vi "MPExxx_Reset.vi"(2 "error in (no error)":errorcluster, 3 "VISA session":refnum<visa-resource-name>) -> (0 "error out":errorcluster, 1 "dup VISA session":refnum<visa-resource-name>)   [LabVIEW 2023]
doc: "This command resets the power supply to factory default states as defined below.\n\n OUTP[:STAT] OFF\n CURR[:LEV][:IMM] 0 \n CURR[:LEV]:TRIG 0 \n VOLT[:LEV][:IMM] 0 \n VOLT[:LEV]:TRIG 0 \n PER 0\n INIT:CONT OFF\n VOLT:PROT[:LEV] 110% of MAX\n CURR:PROT[:LEV] 110% of MAX"
panel:
  # "MAGNA-POWER"
  # "Electronics"
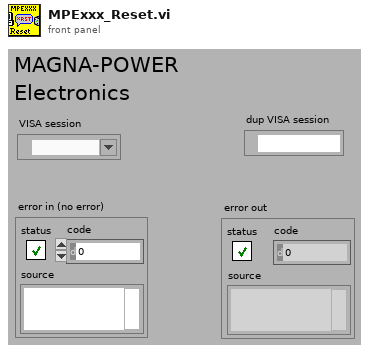
[diagram p1: front panel]
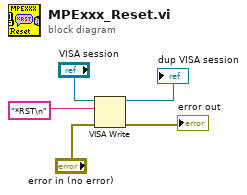
[diagram p0: block diagram]
diagram:
  n1 = VISA Write(VISA resource name="VISA session", write buffer="*RST\n", error in (no error)="error in (no error)") -> (VISA resource name out=→"dup VISA session":refnum<visa-resource-name>, error out=→"error out":errorcluster)  [unwired: 1 out]
